vi "OpenTiffHead.vi"(0 "file path":path, 1 "error in":errorcluster) -> (2 "TIFF file":T2 {"BigTiff,Endian" items=["Big-Endian"=0, "Native"=1, "Little-Endian"=2, "BigTiff-Big-Endian"=256, "Bigtiff,Native"=257, "Biftiff,Littleendian"=258]}, 4 "first Diroffset":u64 format="%.0x", 5 "error out":errorcluster)   [LabVIEW 2011]
panel:
  out "Byte-Reihenfolge":T1(ring)
  out "data":u32 format="%.0x"
  out "First U32":u32 format="%.0x"
  # "Bit 8: BigTiff, Bit0-7 Byte order"
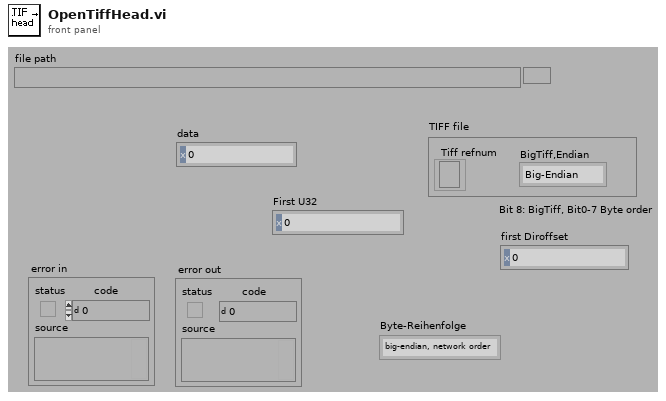
[diagram p1: front panel]
types:
  T1 = enum16{"big-endian, network order", "native, host order", "little-endian", "BigTIFF, big-endian", "BigTIFF, native", "BigTiff, Little-endian"}
  T2 = cluster{"Tiff refnum":refnum<file>, "BigTiff,Endian":u16}
  T3 = enum16{"big-endian, network order", "native, host order", "little-endian"}
  T4 = enum16{"read/write", "read-only", "write-only", "write-only (truncate)"}
  T5 = enum8{"big-endian, network order", "native, host order", "little-endian"}
  T6 = cluster{"refnum out":refnum<file>, "Byte-Reihenfolge (0:Big-Endian, Netzwerkreihenfolge)":u16}
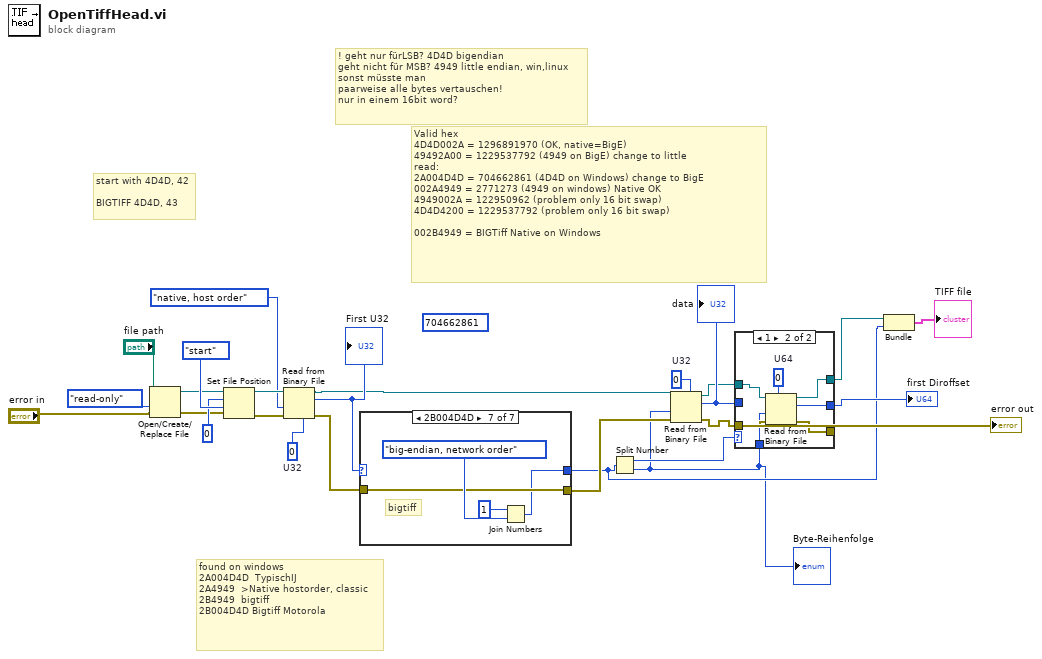
[diagram p0: block diagram]
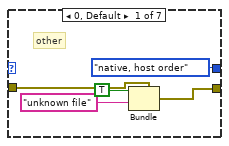
[diagram p3: hidden frame]
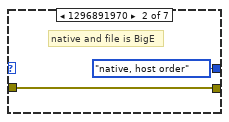
[diagram p4: hidden frame]
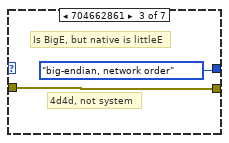
[diagram p5: hidden frame]
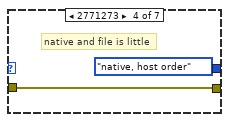
[diagram p6: hidden frame]
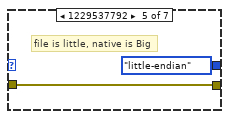
[diagram p7: hidden frame]
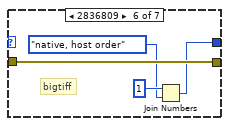
[diagram p8: hidden frame]
diagram:
  w9 = u32 0  # U32
  (unwired) 704662861
  w13 = u32 0  # U32
  # "found on windows\n2A004D4D  TypischIJ\n2A4949  >Native hostorder, classic \n2B4949  bigtiff\n2B004D4D Bigtiff Motorola"
  # "Valid hex\n4D4D002A = 1296891970 (OK, native=BigE)\n49492A00 = 1229537792 (4949 on BigE) change to little \nread:\n2A004D4D = 704662861 (4D4D on Windows) change to BigE\n002A4949 = 2771273 (4949 on windows) Native OK\n4949002A = 122950962 (problem only 16 bit swap)\n4D4D4200 = 1229537792 (problem only 16 bit swap)\n\n002B4949 = BIGTiff Native on Windows"
  # "start with 4D4D, 42\n\nBIGTIFF 4D4D, 43"
  # "! geht nur fürLSB? 4D4D bigendian\ngeht nicht für MSB? 4949 little endian, win,linux\nsonst müsste man \npaarweise alle bytes vertauschen!\nnur in einem 16bit word?"
  n1 = Open/Create/Replace File(file path (use dialog)="file path", error in="error in", access (0:read/write)=T4."read-only" ("open mode (0)")) -> (refnum out=w20:refnum<file>, error out=w19:errorcluster)  [unwired: 4 out]
  n2 = Set File Position(offset (in bytes) (0)=0 ("IFDoffset"), refnum=w20, from (0:start)=enum16{"start", "end", "current"}."start" ("pos mode (0:2)"), error in=w19) -> (refnum out=w18:refnum<file>, error out=w17:errorcluster)
  n3 = Read from Binary File(5:w13, 8:w17, 9:T3."native, host order" ("Byte-Reihenfolge (0:Big-Endian, Netzwerkreihenfolge)"), 11:w18) -> (0:w15:errorcluster, 2:w16:u32, 3:w11:refnum<file>)  [unwired: 3 out]
  "First U32" <- w16
  n4 = case shown="2B004D4D" w16 {
    tunnel: w15 -> [w30 w31 w33 w35 w37 w42 w44]
    tunnel: [w28 w31 w33 w35 w37 w42 w44] -> w12
    tunnel: [T3."native, host order" ("Byte-Reihenfolge (0:Big-Endian, Netzwerkreihenfolge)") T3."native, host order" ("Byte-Reihenfolge (0:Big-Endian, Netzwerkreihenfolge)") T3."big-endian, network order" ("Byte-Reihenfolge (0:Big-Endian, Netzwerkreihenfolge)") T3."native, host order" ("Byte-Reihenfolge (0:Big-Endian, Netzwerkreihenfolge)") T3."little-endian" ("Byte-Reihenfolge (0:Big-Endian, Netzwerkreihenfolge)") w40 w43] -> w2
    frame 0, Default {
      # "other"
      n5 = Bundle(cluster=w30, "status"=TRUE, "source"="unknown file") -> (w28:errorcluster)  [unwired: 1 out]
    }
    frame 1296891970 {
      # "native and file is BigE"
    }
    frame 704662861 {
      # "Is BigE, but native is littleE"
      # "4d4d, not system"
    }
    frame 2771273 {
      # "native and file is little"
    }
    frame 1229537792 {
      # "file is little, native is Big"
    }
    frame 2836809 {
      # "bigtiff"
      n6 = Join Numbers(hi=u8 1, lo=T5."native, host order" ("Byte-Reihenfolge (0:Big-Endian, Netzwerkreihenfolge)")) -> ((hi.lo)=w40:u16)
    }
    frame 721440077 {
      # "bigtiff"
      n7 = Join Numbers(hi=u8 1, lo=T5."big-endian, network order" ("Byte-Reihenfolge (0:Big-Endian, Netzwerkreihenfolge)")) -> ((hi.lo)=w43:u16)
    }
  }
  n8 = Split Number(x=w2) -> (hi(x)=w7:u8, lo(x)=w1:u8)
  "Byte-Reihenfolge" <- w1
  n9 = Read from Binary File(5:w9, 8:w12, 9:w1, 11:w11) -> (0:w8:errorcluster, 2:w6:u32, 3:w4:refnum<file>)  [unwired: 3 out]
  "error out" <- w8
  "data" <- w6
  n10 = case shown="1" w7 {
    tunnel: [w49 w54] -> _
    tunnel: [w48 w52] -> w5
    tunnel: w8 -> [w49 w56]
    tunnel: w6 -> [w48 _]
    tunnel: [w47 w55] -> w3
    tunnel: w4 -> [w47 w50]
    tunnel: w1 -> [_ w51]
    frame 0, Default {
    }
    frame 1 {
      w53 = u64 0  # U64
      n11 = Read from Binary File(5:w53, 8:w56, 9:w51, 11:w50) -> (0:w54:errorcluster, 2:w52:u64, 3:w55:refnum<file>)  [unwired: 3 out]
    }
  }
  "first Diroffset" <- w5
  n12 = Bundle("refnum out"=w3, "Byte-Reihenfolge (0:Big-Endian, Netzwerkreihenfolge)"=w2) -> (→"TIFF file":T6)  [unwired: 1 out]
